vi "svx_Snd Read Waveform.vi"(8 "error in (no error)":errorcluster, 11 "wave file path":path) -> (0 "error out":errorcluster, 2 "Channel 2":waveform(dbl), 3 "Channel 1":waveform(dbl), 4 "SVT WAV info":T1)   [LabVIEW 2017]
doc: "Reads stereo waveform data from WAV file."
uses:
  <vilib>/addons/_NISVFA/_Shared subVIs/Controls/SVT WAV Info.ctl
  <vilib>/addons/_NISVFA/_Shared subVIs/Controls/DAQ Coupling for SVT WAV Info.ctl
  <vilib>/addons/_NISVFA/_Shared subVIs/Controls/DAQ Polarity for SVT WAV Info.ctl
  <vilib>/addons/_NISVFA/_Shared subVIs/Controls/DAQ Terminal Configuration for SVT WAV Info.ctl
panel:
  in  "SVT WAV info":T1
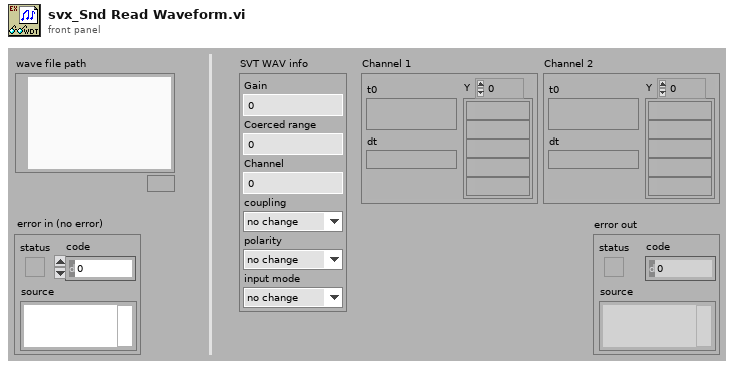
[diagram p1: front panel]
types:
  T1 = typedef "SVT WAV Info.ctl" = cluster{"Gain":u16, "Coerced range":u16, "Channel":u16, "coupling":T2, "polarity":T3, "input mode":T4}
  T2 = typedef "DAQ Coupling for SVT WAV Info.ctl" = enum16{"no change", "DC", "AC", "ground", "internal reference"}
  T3 = typedef "DAQ Polarity for SVT WAV Info.ctl" = enum16{"no change", "bipolar", "unipolar"}
  T4 = typedef "DAQ Terminal Configuration for SVT WAV Info.ctl" = enum16{"no change", "differential", "rse", "nrse", "pseudodifferential"}
  T5 = enum16{"open", "replace", "create", "open or create", "replace or create", "replace or create with confirmation"}
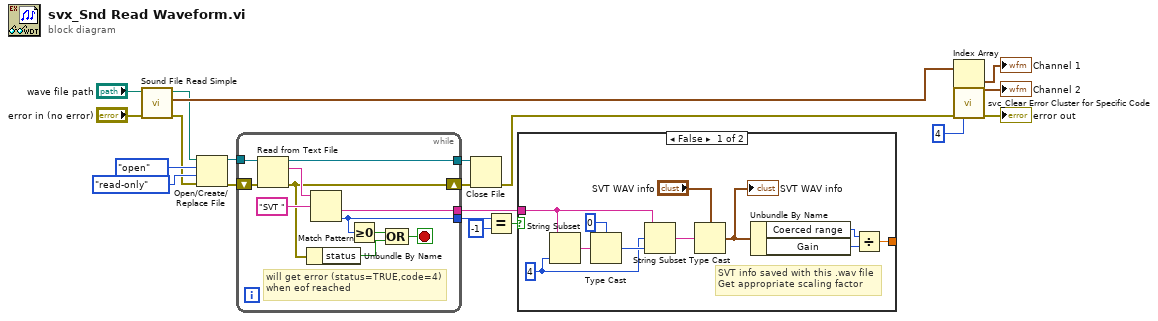
[diagram p0: block diagram]
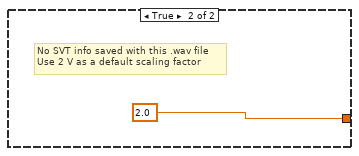
[diagram p2: hidden frame]
diagram:
  n1 = call <vilib>:"Sound File Read Simple.vi"("error in (no error)"="error in (no error)", "path"="wave file path") -> ("error out"=w4:errorcluster, "data"=w15:waveform(dbl)[], "path out"=w7:path)  [unwired: 6 in, 1 out]
  n2 = Open/Create/Replace File(file path (use dialog)=w7, error in=w4, operation (0:open)=T5."open", access (0:read/write)=enum16{"read/write", "read-only", "write-only"}."read-only") -> (refnum out=w14:refnum<file>, error out=w6:errorcluster)  [unwired: 2 in, 1 out]
  n3 = while {
    tunnel: w14 -> [w26]
    tunnel: [w25] -> w10
    tunnel: [w24] -> w11
    tunnel: [w23] -> w9
    shift-right: [w21] -> w5
    shift-left: w6 -> [w22]
    stop <- w28 stop-if-true
    # "will get error (status=TRUE,code=4) when eof reached"
    n4 = Read from Text File(file (use dialog)=w26, error in=w22) -> (refnum out=w23:refnum<file>, text=w31:string, error out=w21:errorcluster)  [unwired: 2 in, 1 out]
    n5 = Unbundle By Name(w21) -> ("status"=w29:bool)
    n6 = Match Pattern(string=w31, regular expression="SVT ") -> (after substring=w24:string, offset past match=w25:i32)  [unwired: 1 in, 2 out]
    n7 = Greater Or Equal To 0?(x=w25) -> (x >= 0?=w27:bool)
    n8 = Compound Arithmetic op=OR(w27, w29) -> (w28:bool)
  }
  n9 = Close File(refnum=w9, error in=w5) -> (error out=w3:errorcluster)  [unwired: 1 out]
  n10 = Equal?(x=w10, y=-1) -> (x = y?=w16:bool)
  n11 = case shown="False" w16 {
    tunnel: w11 -> [w40 _]
    tunnel: [w35 2.0] -> _
    frame False {
      w32 = 4 ("length (rest)")
      (unwired) 4 ("Array Length")
      # "SVT info saved with this .wav file Get appropriate scaling factor"
      n12 = String Subset(string=w40, length (rest)=w32) -> (substring=w42:string)  [unwired: 1 in]
      n13 = Type Cast(type=u32 0, x=w42) -> (*(type *) &x=w39:u32)
      n14 = String Subset(string=w40, offset (0)=w32, length (rest)=w39) -> (substring=w37:string)
      n15 = Type Cast(type="SVT WAV info", x=w37) -> (*(type *) &x=w36:T1)
      "SVT WAV info" <- w36
      n16 = Unbundle By Name(w36) -> ("Coerced range"=w34:u16, "Gain"=w33:u16)
      n17 = Divide(x=w34, y=w33) -> (x/y=w35:dbl)
    }
    frame True {
      # "No SVT info saved with this .wav file\nUse 2 V as a default scaling factor"
    }
  }
  n18 = Index Array(array=w15) -> (element #1=→"Channel 1":waveform(dbl), element #2=→"Channel 2":waveform(dbl))  [unwired: 2 in]
  n19 = call <vilib>:"svc_Clear Error Cluster for Specific Code.vi"("error in (no error)"=w3, "code"=4) -> ("error out"=→"error out":errorcluster)  [unwired: 12 in, 1 out]
